vi "Write Maximum Time.vi"(8 "error in (no error)":errorcluster, 10 "Maximum Time":dbl[unit], 11 "TDMS-Actor in":refnum<class "TDMS-Actor.lvclass">) -> (0 "error out":errorcluster, 3 "TDMS-Actor out":refnum<class "TDMS-Actor.lvclass">)   [LabVIEW 2015, in "BNT_TDMS.lvlib" / "TDMS-Actor.lvclass"]
doc: "Write maxium time for file change to attribute."
uses:
  TDMS-Actor.lvclass
  TDMS-Actor.lvclass/TDMS-Actor.ctl
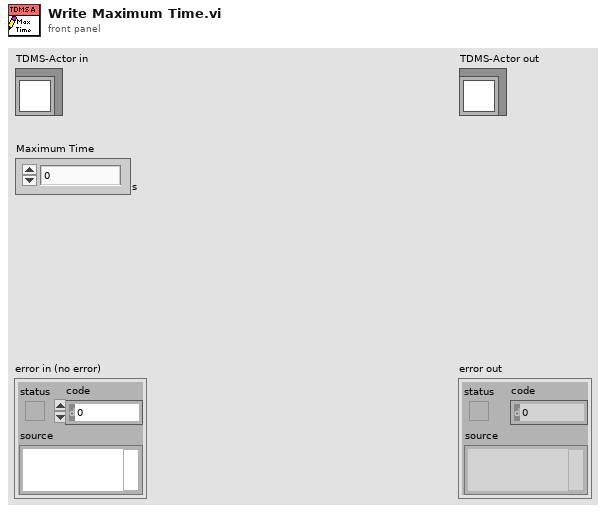
[diagram p1: front panel]
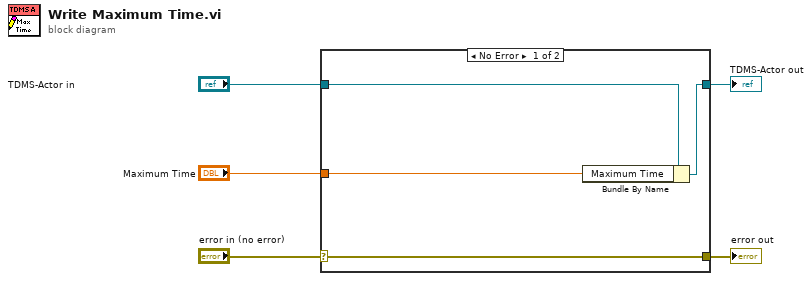
[diagram p0: block diagram]
diagram:
  n1 = case shown="No Error" "error in (no error)" {
    selector: "error in (no error)" -> [w9 w10]
    tunnel: [w9 w10] -> w4
    tunnel: [w7 w11] -> w2
    tunnel: "TDMS-Actor in" -> [w8 w11]
    tunnel: "Maximum Time" -> [w6 _]
    frame No Error {
      n2 = Bundle By Name(cluster=w8, "Maximum Time"=w6) -> (w7:refnum<class "TDMS-Actor.lvclass">)
    }
    frame Error {
    }
  }
  "error out" <- w4
  "TDMS-Actor out" <- w2
